vi "Broadcast Response.vi"(8 "error in (no error)":errorcluster, 9 "Acquired Result.lvclass":refnum<class "Acquired Result.lvclass">, 10 "Topic":string, 11 "Lockin Processor in":refnum<class "Lockin Processor.lvclass">) -> (0 "error out":errorcluster, 3 "Lockin Processor out":refnum<class "Lockin Processor.lvclass">)   [LabVIEW 2015, in "Lockin Processor.lvclass"]
uses:
  Lockin Processor.lvclass
  Measure_core/Results/Acquired Result/Acquired Result.lvclass
  Read Lockin Processor Configuration.vi
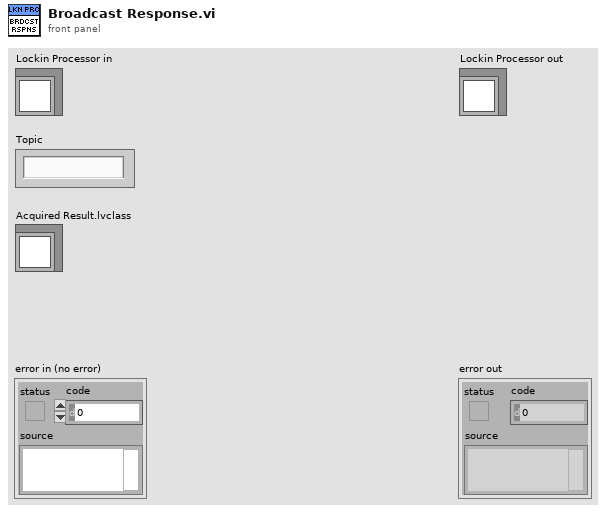
[diagram p1: front panel]
types:
  T1 = typedef "Lockin Processor Configuration.ctl" = cluster{"Time constant":dbl, "Phase":dbl, "Signal channels":string[], "Group":string, "Clip units of Ts off":dbl, "X channel":string}
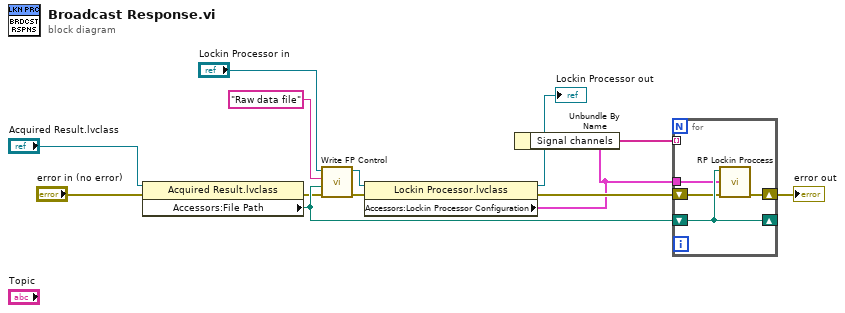
[diagram p0: block diagram]
diagram:
  n1 = property class="Acquired Result.lvclass"(reference="Acquired Result.lvclass", error in="error in (no error)") -> (error out=w4:errorcluster, "Accessors:File Path"=w5:path)  [unwired: 1 out]
  n2 = call-dynamic "Write FP Control.vi"("error in (no error)"=w4, "Control Value"=w5, "Control Name"="Raw data file", "Measure Object in"="Lockin Processor in") -> ("error out"=w3:errorcluster, "Measure Object out"=w7:refnum<class "Lockin Processor.lvclass">)  [unwired: 6 in]
  n3 = property class="Lockin Processor.lvclass"(reference=w7, error in=w3) -> (reference out=→"Lockin Processor out":refnum<class "Lockin Processor.lvclass">, error out=w10:errorcluster, "Accessors:Lockin Processor Configuration"=w2:T1)
  n4 = Unbundle By Name(w2) -> ("Signal channels"=w1:string[])
  n5 = for {
    shift-right: [w17] -> _
    shift-left: w5 -> [w17]
    shift-right: [w15] -> w9
    shift-left: w10 -> [w16]
    tunnel: w2 -> [w14]
    tunnel: w1 -> [_] mode=indexing
    n6 = call "RP Lockin Proccess.vi"("Error In"=w16, "Configuration"=w14, "Signal file"=w17) -> ("Error Out"=w15:errorcluster)  [unwired: 8 in]
  }
  "error out" <- w9
